vi "RT DAQ v2.vi"() -> ()   [LabVIEW 2024]
uses:
  Ramps.ctl
  <vilib>/FPGAPlugInAG/cRIO-9063/niLvFpga_Open_cRIO-9063.vi
  <vilib>/rvi/interface/common/dynamic/niFpgaDynamicAddResources.vi
  <vilib>/FPGAPlugInAG/Dynamic/niLvFpga_Reset_Dynamic.vi
  <vilib>/FPGAPlugInAG/Dynamic/niLvFpga_Run_Dynamic.vi
  <vilib>/Utility/error.llb/Error Cluster From Error Code.vi
  <vilib>/rvi/errors/niLvFpgaAdjustHostInterfaceError.vi
  <vilib>/FPGAPlugInAG/Dynamic/niLvFpga_Close_Dynamic.vi
  <vilib>/FPGAPlugInAG/Dynamic/niLvFpga_Abort_Dynamic.vi
  <vilib>/RVI Host/nirviSupport.llb/nirviErrorClusterFromErrorCode.vi
  <vilib>/rvi/interface/nirviOpenFPGA/nirviOpenFPGA.xnode
  Transport measurement/FPGA Bitfiles/Mainproject_FPGATarget_SinglepointDAQ2_KFK63D1NkjA.lvbitx
  simple DAQ.vi
  <vilib>/rvi/interface/nirviMethod/nirviMethod.xnode
  <vilib>/rvi/interface/nirviReadWriteControl/nirviReadWriteControl.xnode
  <vilib>/rvi/interface/nirviCloseFPGA/nirviCloseFPGA.xnode
  Transport measurement/FPGA Bitfiles/transportmain_FPGATarget_AWGIVmeasurement_k024ycvYU0o.lvbitx
  AWG IV measurement.vi
  <vilib>/rvi/interface/nirviMethod/StockFPGA_InlinedMethodWaitForSingleIRQ.vi
  <vilib>/FPGAPlugInAG/Dynamic/niLvFpga_WaitOnIrq_Dynamic.vi
  <vilib>/FPGAPlugInAG/Dynamic/niLvFpga_AcknowledgeIrq_Dynamic.vi
  <vilib>/rvi/interface/Simulation/niFpgaSimulationCallBeginRW.vi
  <vilib>/NI_Real-Time Target Support.lvlib
  NiFpgaLv.dll
panel:
  out "AWG test parameter":T1={"Amp"=0.0, "Delay time 10us"=100, "Ramp1 time 10us"=1000, "Ramp2 time 10us"=2000, "Ramp3 time 10us"=1000, "End time 10us"=200}
  out "FPGA DAQ1":refnum<k20>
  out "FPGA DAQ":refnum<k20>
  out "VI Stop":bool
  out "error out":errorcluster
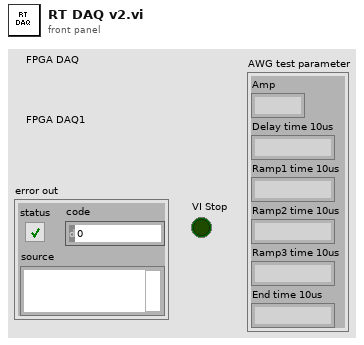
[diagram p1: front panel]
types:
  T1 = typedef "Ramps.ctl" = cluster{"Amp":fxp<+/-,20,5>, "Delay time 10us":i32, "Ramp1 time 10us":i32, "Ramp2 time 10us":i32, "Ramp3 time 10us":i32, "End time 10us":i32}
  T2 = cluster{"Command":string, "Voltage":dbl, "Channel":string}
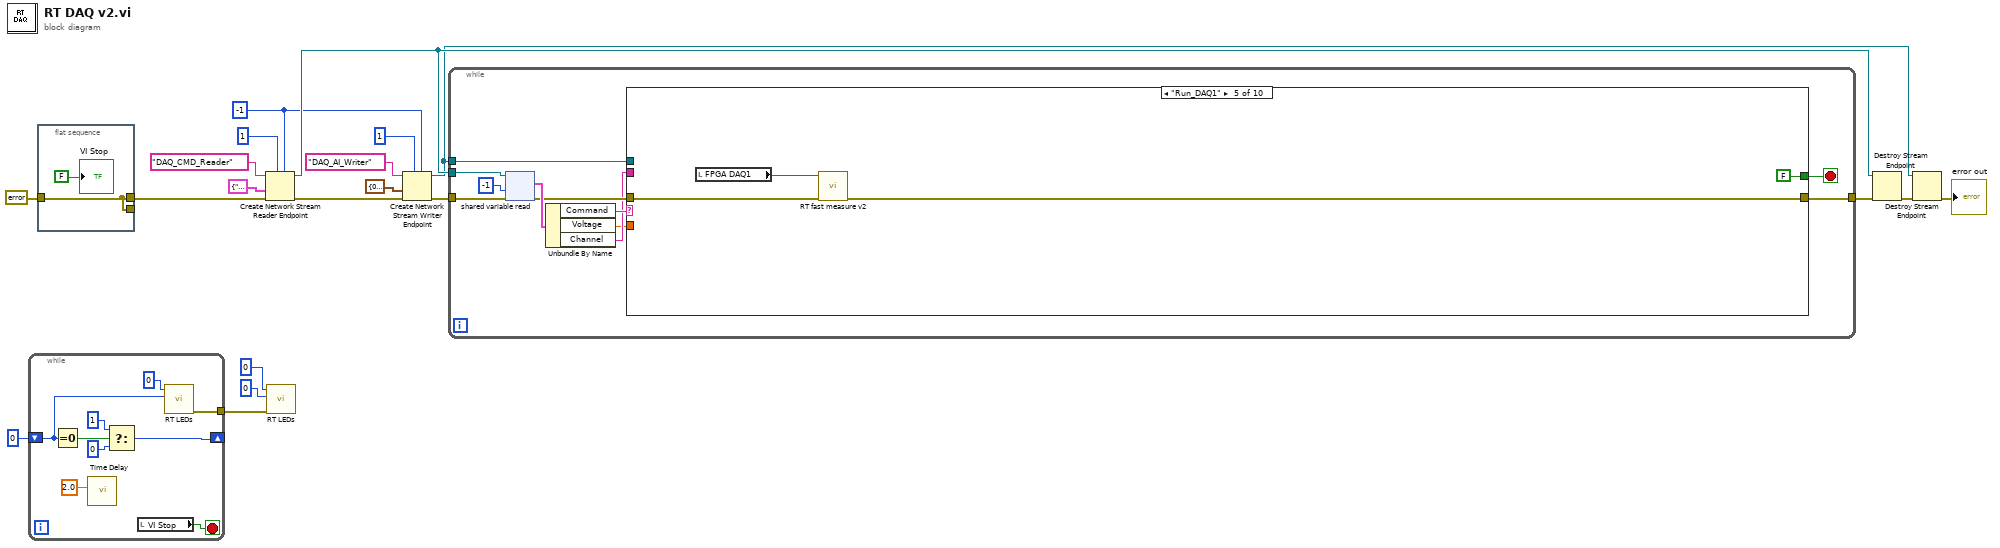
[diagram p0: block diagram]
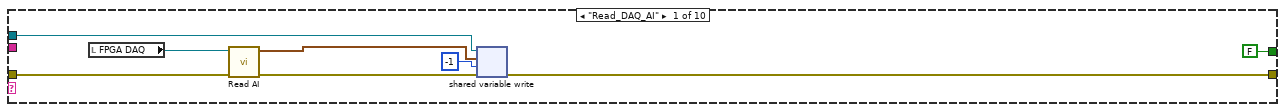
[diagram p2: hidden frame]
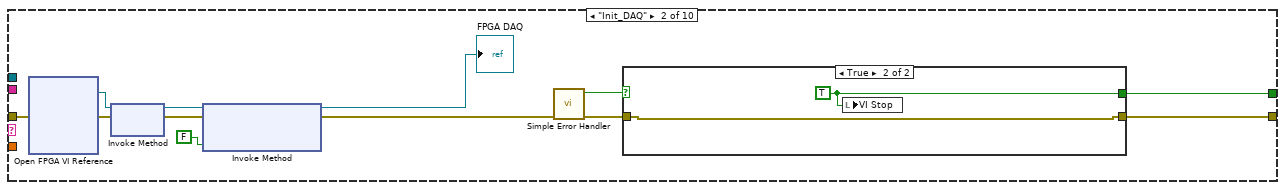
[diagram p3: hidden frame]
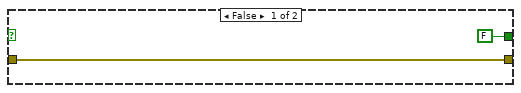
[diagram p4: hidden frame]
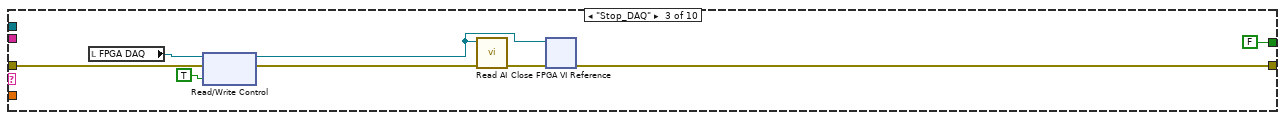
[diagram p5: hidden frame]
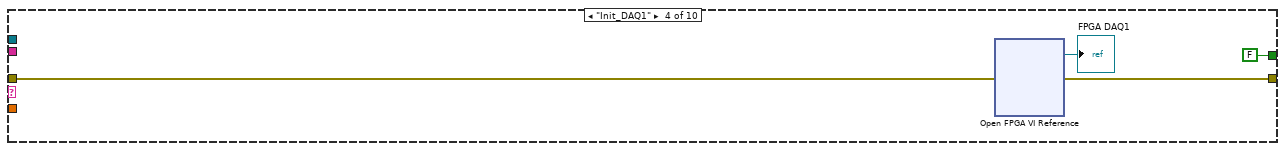
[diagram p6: hidden frame]
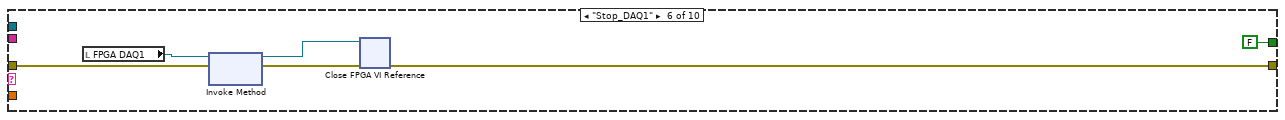
[diagram p7: hidden frame]
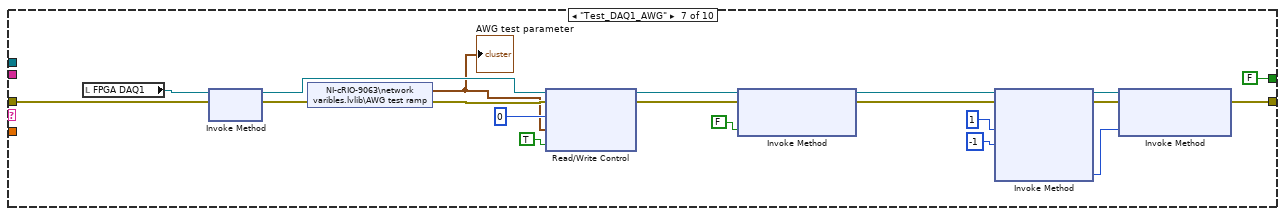
[diagram p8: hidden frame]
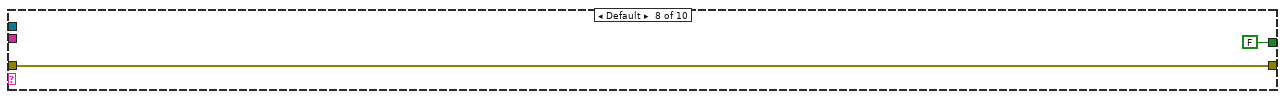
[diagram p9: hidden frame]
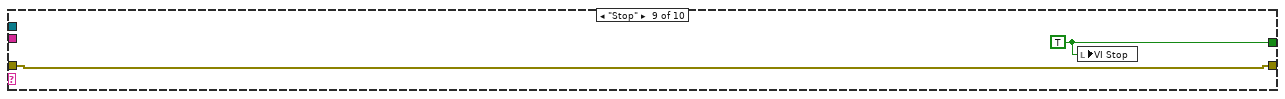
[diagram p10: hidden frame]
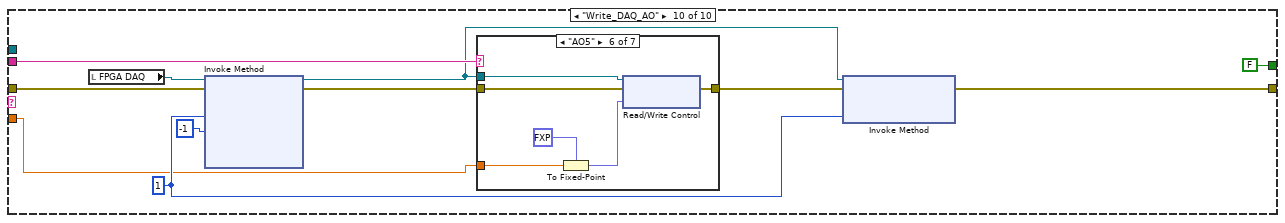
[diagram p11: hidden frame]
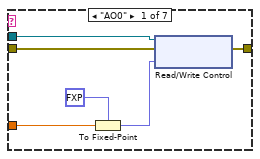
[diagram p12: hidden frame]
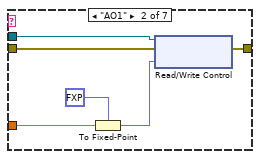
[diagram p13: hidden frame]
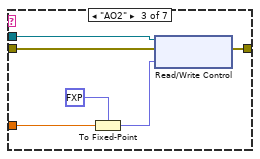
[diagram p14: hidden frame]
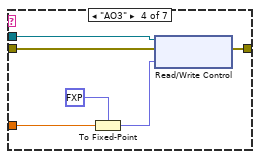
[diagram p15: hidden frame]
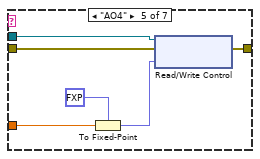
[diagram p16: hidden frame]
diagram:
  w3 = -1 ("timeout in ms (-1)")
  n1 = while {
    shift-right: [w24] -> _
    shift-left: 0 ("State") -> [w28]
    tunnel: [w21] -> w5
    stop <- w22 stop-if-true
    n2 = Equal To 0?(x=w28) -> (x = 0?=w27:bool)
    n3 = call "Time Delay"("Delay Time (s)"=2.0) -> ()  [unwired: 10 in, 1 out]
    n4 = Select(t=1, s=w27, f=0) -> (s? t:f=w24:i32)
    n5 = local read "VI Stop"() -> (w22:bool)
    n6 = call <vilib>:"RT LEDs.vi"("State"=w28, "LED Num"=0) -> ("error out"=w21:errorcluster)  [unwired: 4 in, 1 out]
  }
  n7 = flat-sequence {
    tunnel: errorcluster {"status"=FALSE, "code"=0, "source"=""} ("error in (no error)") -> [w30]
    tunnel: [w30] -> _
    tunnel: [w30] -> w2
    frame #0 {
      "VI Stop" <- FALSE ("VI Stop")
    }
  }
  n8 = Create Network Stream Reader Endpoint(5:w3, 7:1 ("reader buffer size"), 8:w2, 9:T2 {"Command"="", "Voltage"=0.0, "Channel"=""} ("Write cluster"), 11:"DAQ_CMD_Reader" ("reader name")) -> (0:w12:errorcluster, 3:w17:refnum<k21>)  [unwired: 2 in]
  n9 = call <vilib>:"RT LEDs.vi"("error in (no error)"=w5, "State"=0, "LED Num"=0) -> ()  [unwired: 3 in, 2 out]
  n10 = Create Network Stream Writer Endpoint(5:w3, 7:1 ("writer buffer size"), 8:w12, 9:cluster{dbl, dbl, dbl, dbl} {0.0, 0.0, 0.0, 0.0} ("output cluster"), 11:"DAQ_AI_Writer" ("reader name")) -> (0:w9:errorcluster, 3:w11:refnum<k21>)  [unwired: 2 in]
  n11 = while {
    tunnel: w9 -> [w42]
    tunnel: w17 -> [w41]
    tunnel: [w33] -> w18
    tunnel: w11 -> [w34]
    stop <- w32 stop-if-true
    n12 = shared-variable-read(w41, w42, -1 ("timeout ms (-1)")) -> (w37:errorcluster, w39:T2)  [unwired: 2 out]
    n13 = Unbundle By Name(w39) -> ("Command"=w38:string, "Voltage"=w35:dbl, "Channel"=w36:string)
    n14 = case shown="\"Run_DAQ1\"" w38 {
      tunnel: w37 -> [w50 w57 w72 w75 w82 w85 w105 w109 w112 w120]
      tunnel: w36 -> [_ _ _ _ _ _ _ _ _ w118]
      tunnel: w35 -> [_ _ _ _ _ _ _ _ _ w117]
      tunnel: [w45 w53 w68 w78 w79 w88 w98 w109 w112 w116] -> w33
      tunnel: w34 -> [w49 _ _ _ _ _ _ _ _ _]
      tunnel: [FALSE w54 FALSE FALSE FALSE FALSE FALSE FALSE w111 FALSE] -> w32
      frame "Read_DAQ_AI" {
        n15 = local read "FPGA DAQ"() -> (w43:refnum<k20>)
        n16 = call "Read AI.vi"("error in (no error)"=w50, "Refnum in"=w43) -> ("error out"=w47:errorcluster, "data"=w48:cluster{dbl, dbl, dbl, dbl})  [unwired: 8 in]
        n17 = shared-variable-write(w49, w47, w48, -1 ("timeout ms (-1)")) -> (w45:errorcluster)  [unwired: 2 out]
      }
      frame "Init_DAQ" {
        n18 = xnode "Open FPGA VI Reference"("error in"=w57) -> ("FPGA VI Reference Out"=w60:refnum<k20>, "error out"=w61:errorcluster)  [unwired: 1 in]
        n19 = xnode "Invoke Method"("FPGA VI Reference In"=w60, "error in"=w61) -> ("FPGA VI Reference Out"=w59:refnum<k20>, "error out"=w62:errorcluster)
        n20 = xnode "Invoke Method"("FPGA VI Reference In"=w59, "error in"=w62, "Wait Until Done (F)"=FALSE) -> ("FPGA VI Reference Out"=→"FPGA DAQ":refnum<k20>, "error out"=w56:errorcluster)
        n21 = call <vilib>:"Simple Error Handler.vi"("error in (no error)"=w56) -> ("error?"=w55:bool, "error out"=w52:errorcluster)  [unwired: 4 in, 3 out]
        n22 = case shown="True" w55 {
          tunnel: [FALSE w65] -> w54
          tunnel: [w63 w66] -> w53
          tunnel: w52 -> [w63 w66]
          frame False {
          }
          frame True {
            w65 = TRUE
            n23 = local write "VI Stop"(w65) -> ()
          }
        }
      }
      frame "Stop_DAQ" {
        n24 = local read "FPGA DAQ"() -> (w73:refnum<k20>)
        n25 = xnode "Read/Write Control"("FPGA VI Reference In"=w73, "error in"=w72, "Stop"=TRUE) -> ("FPGA VI Reference Out"=w67:refnum<k20>, "error out"=w70:errorcluster)
        n26 = call "Read AI.vi"("error in (no error)"=w70, "Refnum in"=w67) -> ("error out"=w69:errorcluster)  [unwired: 8 in, 1 out]
        n27 = xnode "Close FPGA VI Reference"("FPGA VI Reference In"=w67, "error in"=w69) -> ("error out"=w68:errorcluster)
      }
      frame "Init_DAQ1" {
        n28 = xnode "Open FPGA VI Reference"("error in"=w75) -> ("FPGA VI Reference Out"=→"FPGA DAQ1":refnum<k20>, "error out"=w78:errorcluster)  [unwired: 1 in]
      }
      frame "Run_DAQ1" {
        n29 = local read "FPGA DAQ1"() -> (w80:refnum<k20>)
        n30 = call "RT fast measure v2.vi"("error in"=w82, "FPGA DAQ1"=w80) -> ("error out"=w79:errorcluster)  [unwired: 9 in]
      }
      frame "Stop_DAQ1" {
        n31 = local read "FPGA DAQ1"() -> (w86:refnum<k20>)
        n32 = xnode "Invoke Method"("FPGA VI Reference In"=w86, "error in"=w85) -> ("FPGA VI Reference Out"=w83:refnum<k20>, "error out"=w84:errorcluster)
        n33 = xnode "Close FPGA VI Reference"("FPGA VI Reference In"=w83, "error in"=w84) -> ("error out"=w88:errorcluster)
      }
      frame "Test_DAQ1_AWG" {
        n34 = local read "FPGA DAQ1"() -> (w106:refnum<k20>)
        n35 = xnode "Invoke Method"("FPGA VI Reference In"=w106, "error in"=w105) -> ("FPGA VI Reference Out"=w93:refnum<k20>, "error out"=w91:errorcluster)
        n36 = shared-variable "NI-cRIO-9063\\network varibles.lvlib\\AWG test ramp"(error in=w91) -> (w89:T1, error out=w90:errorcluster)
        "AWG test parameter" <- w89
        n37 = xnode "Read/Write Control"("FPGA VI Reference In"=w93, "error in"=w90, "Records Num"=0, "Ramps"=w89, "Init gate"=TRUE) -> ("FPGA VI Reference Out"=w95:refnum<k20>, "error out"=w94:errorcluster)
        n38 = xnode "Invoke Method"("FPGA VI Reference In"=w95, "error in"=w94, "Wait Until Done (F)"=FALSE) -> ("FPGA VI Reference Out"=w97:refnum<k20>, "error out"=w96:errorcluster)
        n39 = xnode "Invoke Method"("FPGA VI Reference In"=w97, "error in"=w96, "IRQ Number(s)"=1, "Timeout (ms)"=-1) -> ("FPGA VI Reference Out"=w101:refnum<k20>, "error out"=w100:errorcluster, "IRQ(s) Asserted"=w99:i32)  [unwired: 1 out]
        n40 = xnode "Invoke Method"("FPGA VI Reference In"=w101, "error in"=w100, "IRQ Number(s)"=w99) -> ("error out"=w98:errorcluster)  [unwired: 1 out]
      }
      frame Default {
      }
      frame "Stop" {
        w111 = TRUE
        n41 = local write "VI Stop"(w111) -> ()
      }
      frame "Write_DAQ_AO" {
        w121 = 1 ("IRQ Number(s)")
        n42 = local read "FPGA DAQ"() -> (w113:refnum<k20>)
        n43 = xnode "Invoke Method"("FPGA VI Reference In"=w113, "error in"=w120, "IRQ Number(s)"=w121, "Timeout (ms)"=-1) -> ("FPGA VI Reference Out"=w114:refnum<k20>, "error out"=w122:errorcluster)  [unwired: 2 out]
        n44 = case shown="\"AO5\"" w118 {
          tunnel: w114 -> [w129 w133 w139 w145 w151 w157 _]
          tunnel: w117 -> [w126 w131 w138 w144 w149 w155 _]
          tunnel: w122 -> [w125 w132 w137 w143 w150 w156 w160]
          tunnel: [w124 w130 w136 w142 w148 w154 w160] -> w123
          frame "AO0" {
            n45 = To Fixed-Point(fixed-point type=fxp<+/-,20,5> 0.0 ("Mod3/AO0"), number=w126) -> (fixed-point=w127:fxp<+/-,20,5>)
            n46 = xnode "Read/Write Control"("FPGA VI Reference In"=w129, "error in"=w125, "Mod3/AO0"=w127) -> ("error out"=w124:errorcluster)  [unwired: 1 out]
          }
          frame "AO1" {
            n47 = To Fixed-Point(fixed-point type=fxp<+/-,20,5> 0.0 ("Mod3/AO0"), number=w131) -> (fixed-point=w134:fxp<+/-,20,5>)
            n48 = xnode "Read/Write Control"("FPGA VI Reference In"=w133, "error in"=w132, "Mod3/AO1"=w134) -> ("error out"=w130:errorcluster)  [unwired: 1 out]
          }
          frame "AO2" {
            n49 = To Fixed-Point(fixed-point type=fxp<+/-,20,5> 0.0 ("Mod3/AO0"), number=w138) -> (fixed-point=w140:fxp<+/-,20,5>)
            n50 = xnode "Read/Write Control"("FPGA VI Reference In"=w139, "error in"=w137, "Mod3/AO2"=w140) -> ("error out"=w136:errorcluster)  [unwired: 1 out]
          }
          frame "AO3" {
            n51 = To Fixed-Point(fixed-point type=fxp<+/-,20,5> 0.0 ("Mod3/AO0"), number=w144) -> (fixed-point=w146:fxp<+/-,20,5>)
            n52 = xnode "Read/Write Control"("FPGA VI Reference In"=w145, "error in"=w143, "Mod3/AO3"=w146) -> ("error out"=w142:errorcluster)  [unwired: 1 out]
          }
          frame "AO4" {
            n53 = To Fixed-Point(fixed-point type=fxp<+/-,20,5> 0.0 ("Mod3/AO0"), number=w149) -> (fixed-point=w152:fxp<+/-,20,5>)
            n54 = xnode "Read/Write Control"("FPGA VI Reference In"=w151, "error in"=w150, "Mod3/AO4"=w152) -> ("error out"=w148:errorcluster)  [unwired: 1 out]
          }
          frame "AO5" {
            n55 = To Fixed-Point(fixed-point type=fxp<+/-,20,5> 0.0 ("Mod3/AO0"), number=w155) -> (fixed-point=w158:fxp<+/-,20,5>)
            n56 = xnode "Read/Write Control"("FPGA VI Reference In"=w157, "error in"=w156, "Mod3/AO5"=w158) -> ("error out"=w154:errorcluster)  [unwired: 1 out]
          }
          frame Default {
          }
        }
        n57 = xnode "Invoke Method"("FPGA VI Reference In"=w114, "error in"=w123, "IRQ Number(s)"=w121) -> ("error out"=w116:errorcluster)  [unwired: 1 out]
      }
    }
  }
  n58 = Destroy Stream Endpoint(8:w18, 11:w17) -> (0:w16:errorcluster)
  n59 = Destroy Stream Endpoint(8:w16, 11:w11) -> (0:→"error out":errorcluster)
